vi "Double Float LT.vi"(11 "Data In":dbl) -> (3 "Data Out":dbl)   [LabVIEW 2016]
uses:
  Core/Assert API Components/Failure Actions.ctl
  Core/Assert API Components/VI References.ctl
  Core/Assert API Components/Assert API Components.lvlib
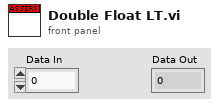
[diagram p1: front panel]
types:
  T1 = typedef "Assert API Components.lvlib/VI References.ctl" = cluster{"Calling VI Ref":refnum<vi>, "Assert VI Ref":refnum<vi>}
  T2 = typedef "Assert API Components.lvlib/Failure Actions.ctl" = enum16{"None", "Log To File", "Pause Execution", "Abort Execution"}
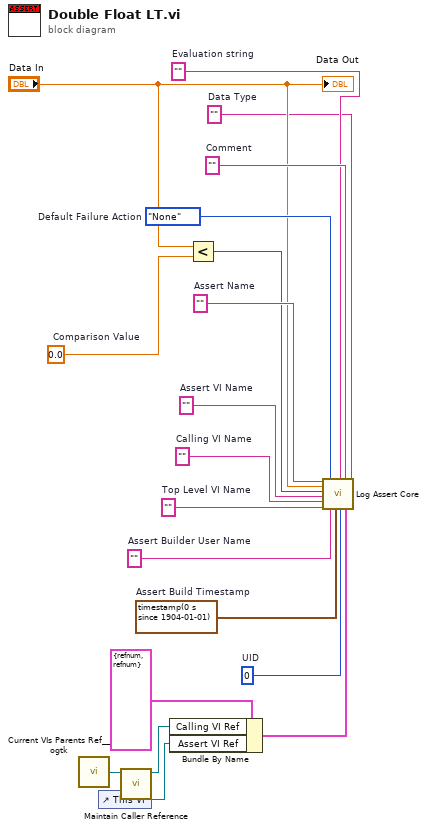
[diagram p0: block diagram]
diagram:
  w2 = ""  # Top Level VI Name
  w3 = 0  # UID
  w4 = ""  # Assert VI Name
  w5 = ""  # Calling VI Name
  w6 = ""  # Data Type
  w7 = ""  # Assert Builder User Name
  w8 = timestamp(0 s since 1904-01-01)  # Assert Build Timestamp
  w16 = ""  # Comment
  w13 = ""  # Evaluation string
  w18 = Failure_Actions."None"  # Default Failure Action
  w19 = ""  # Assert Name
  w17 = 0.0  # Comparison Value
  n1 = call <userlib>:"Current VIs Parents Ref__ogtk.vi"() -> ("Calling VI's Reference"=w11:refnum<vi>)  [unwired: 2 in]
  n2 = control-ref of="This VI"() -> (w10:refnum<vi>)
  n3 = call "Maintain Caller Reference.vi"("VI in"=w11) -> ("VI out"=w1:refnum<vi>)  [unwired: 10 in]
  n4 = Bundle By Name(cluster=T1 {"Calling VI Ref"=refnum, "Assert VI Ref"=refnum} ("VI References"), "Calling VI Ref"=w1, "Assert VI Ref"=w10) -> (w9:T1)
  n5 = Less?(x="Data In", y=w17) -> (x < y?=w14:bool)
  n6 = call "Log Assert Core.vi"("Assert Name"=w19, "Data Value"="Data In", "Status"=w14, "Assert VI Name"=w4, "Calling VI Name"=w5, "Top Level VI Name"=w2, "Failure Action"=w18, "Assert Builder User Name"=w7, "Assert Build Timestamp"=w8, "Evaluation String"=w13, "Assert VI UID"=w3, "Comment"=w16, "VI References"=w9, "Data Type"=w6) -> ()  [unwired: 6 in]
  "Data Out" <- "Data In"
